vi "Write Size.vi"(8 "error in (no error)":errorcluster, 10 "Size":i32, 11 "Hesitant Wolf in":refnum<class "Hesitant Wolf.lvclass">) -> (0 "error out":errorcluster, 3 "Hesitant Wolf out":refnum<class "Hesitant Wolf.lvclass">)   [LabVIEW 2015, in "Hesitant Wolf.lvclass"]
uses:
  Hesitant Wolf.lvclass
  Hesitant Wolf.lvclass/Hesitant Wolf.ctl
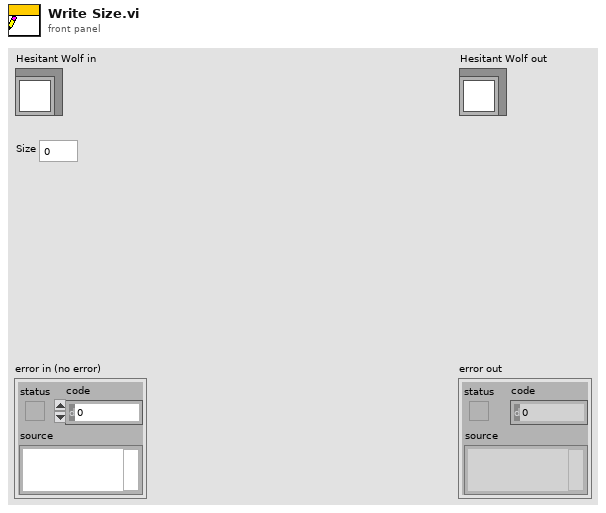
[diagram p1: front panel]
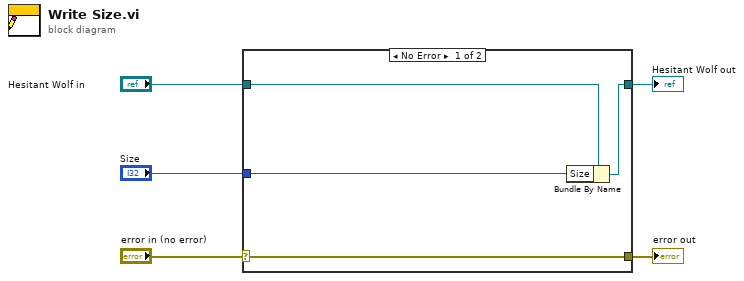
[diagram p0: block diagram]
diagram:
  n1 = case shown="No Error" "error in (no error)" {
    selector: "error in (no error)" -> [w9 w10]
    tunnel: [w9 w10] -> w4
    tunnel: [w7 w11] -> w2
    tunnel: "Hesitant Wolf in" -> [w8 w11]
    tunnel: "Size" -> [w6 _]
    frame No Error {
      n2 = Bundle By Name(cluster=w8, "Size"=w6) -> (w7:refnum<class "Hesitant Wolf.lvclass">)
    }
    frame Error {
    }
  }
  "error out" <- w4
  "Hesitant Wolf out" <- w2
